vi "XY Go.vi"(6 "return immediately":bool, 8 "error in (no error)":errorcluster, 9 "Speed":dbl, 10 "XY In":dbl[](array[numeric]), 11 "Gantry In":refnum<k24>) -> (0 "error out":errorcluster, 2 "XY Out":dbl[](array[numeric]), 3 "Gantry Out":refnum<k24>)   [LabVIEW 2018, in "A3200.lvclass"]
uses:
  A3200.lvclass
  C:/Program Files (x86)/Aerotech/A3200/LabVIEW/2010/Bin/Aerotech.A3200.dll
  Program Files (x86)/Aerotech/A3200/LabVIEW/2010/Bin/Aerotech.A3200.dll
  Drivers/Aerotech A3200/Aerotech.lvlib
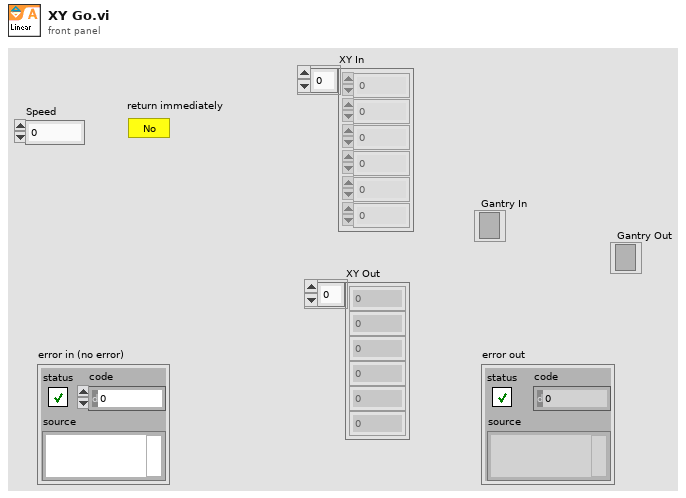
[diagram p1: front panel]
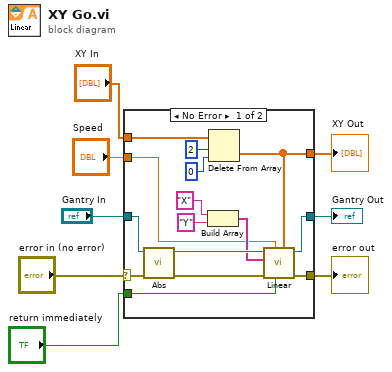
[diagram p0: block diagram]
diagram:
  n1 = case shown="No Error" "error in (no error)" {
    selector: "error in (no error)" -> [w18 w26]
    tunnel: [w16 w26] -> w7
    tunnel: [w20 w25] -> w5
    tunnel: "Gantry In" -> [w19 w25]
    tunnel: "return immediately" -> [w14 _]
    tunnel: [w9 w24] -> w3
    tunnel: "XY In" -> [w12 w24]
    tunnel: "Speed" -> [w13 _]
    frame No Error {
      n2 = call "Abs.vi"("error in (no error)"=w18, "controller in"=w19) -> ("error out"=w17:errorcluster, "controller out"=w21:refnum<k24>)  [unwired: 8 in]
      n3 = Build Array("X" ("format string"), "Y" ("format string")) -> (w15:string[])
      n4 = Delete From Array(array=w12, length=2, index=0) -> (deleted portion=w9:dbl[])  [unwired: 1 out]
      n5 = call "Linear.vi"("distances"=w9, "return immediately"=w14, "speed"=w13, "error in (no error)"=w17, "axis names"=w15, "controller in"=w21) -> ("error out"=w16:errorcluster, "controller out"=w20:refnum<k24>)  [unwired: 4 in]
    }
    frame Error {
    }
  }
  "error out" <- w7
  "Gantry Out" <- w5
  "XY Out" <- w3
